vi "TW Update Supporting Projects.vi"(8 "error in (no error)":errorcluster, 10 "New Name":string, 11 "Template Project Path":path) -> (0 "error out":errorcluster)   [LabVIEW 2021, in "Plugin Generator.lvlib"]
uses:
  Plugin Generator.lvlib
  <vilib>/CIF Foundation/CIF LabVIEW Scripting/LV Scripting/LV Scripting Utilities.lvlib
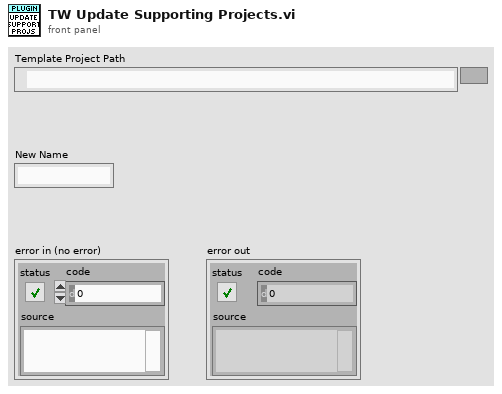
[diagram p1: front panel]
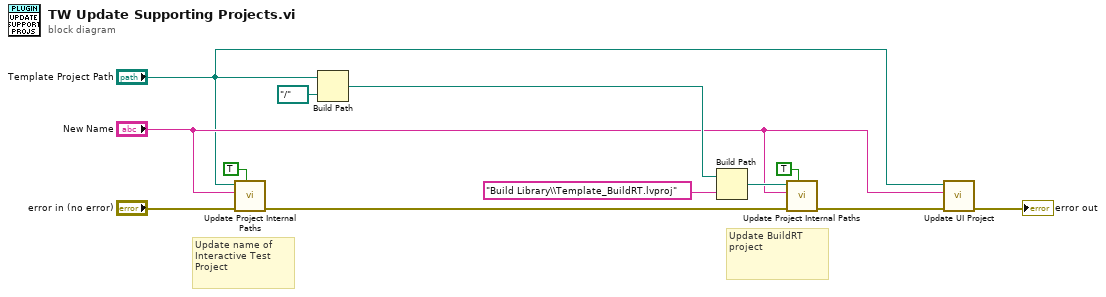
[diagram p0: block diagram]
diagram:
  # "Update BuildRT project"
  # "Update name of Interactive Test Project"
  n1 = call <vilib>:"Update Project Internal Paths.vi"("Rename Project"=TRUE, "error in (no error)"="error in (no error)", "New Subname"="New Name", "Project Path"="Template Project Path") -> ("error out"=w1:errorcluster)  [unwired: 7 in]
  n2 = Build Path(base path="Template Project Path", name or relative path=path "../..") -> (appended path=w7:path)
  n3 = Build Path(base path=w7, name or relative path="Build Library\\Template_BuildRT.lvproj" ("Class Name")) -> (appended path=w9:path)
  n4 = call <vilib>:"Update Project Internal Paths.vi"("Rename Project"=TRUE, "error in (no error)"=w1, "New Subname"="New Name", "Project Path"=w9) -> ("error out"=w5:errorcluster)  [unwired: 7 in]
  n5 = call "Update UI Project.vi"("error in (no error)"=w5, "New Name"="New Name", "Template Project Path"="Template Project Path") -> ("error out"=→"error out":errorcluster)  [unwired: 8 in]
